vi "Extras.vi"(8 "Scope+Safety":T2={"Safety First"={"lim reset"=FALSE, "no limit"=FALSE, "pos slew rate * dt"=100, "neg slew rate * dt"=-100, "Count(Ticks)"=0}, "Scope IPs"={"Trigger Direction"=enum."minus-plus", "Trigger Delay (ms)"=0.0, "Aquisition Rate (kHz)"=4000.0, "Trigger Offset (V)"=0.0, "Scale Offset"={"Scaling"={"Error signal"=1, "Output"=1, "DC Monitor"=1, "Threshold"=1}, "Offset"={"Error Signal"=0, "Output"=0, "DC Monitor"=0, "Threshold"=0}}}}, 11 "Cavity Extras":T3={"Pre-Offset"={"OPO A"=0.0, "OPO B"=0.0, "MCC"=0.0, "Doubler"=0.0}, "Pre-Offset DC"={"OPO A"=0.0, "OPO B"=0.0, "MCC"=0.0, "Doubler"=0.0}, "I Max value"=20000, "I2 Max value"=20000, "Scan Offset"={"OPO A"=0.0, "OPO B"=0.0, "MCC"=0.0, "Doubler"=0.0}, "Scan Ampl."={"OPO A"=1000.0, "OPO B"=1000.0, "MCC"=1000.0, "Doubler"=1000.0}, "Scan-PII thresh"={"OPO A"=0, "OPO B"=0, "MCC"=0, "Doubler"=0}, "Re-Scan thresh"={"OPO A"=0, "OPO B"=0, "MCC"=0, "Doubler"=0}}) -> (0 "Extras Doubler":T1, 1 "Extras MCC":T1, 2 "Extras B":T1, 3 "Extras A":T1)   [LabVIEW 2010]
uses:
  Strict Type Defs/Cavity Extras.ctl
  Strict Type Defs/Pre-Offset.ctl
  Strict Type Defs/Scope and Safety.ctl
  Strict Type Defs/Extras PII.ctl
panel:
  in  "Extras PII":T1
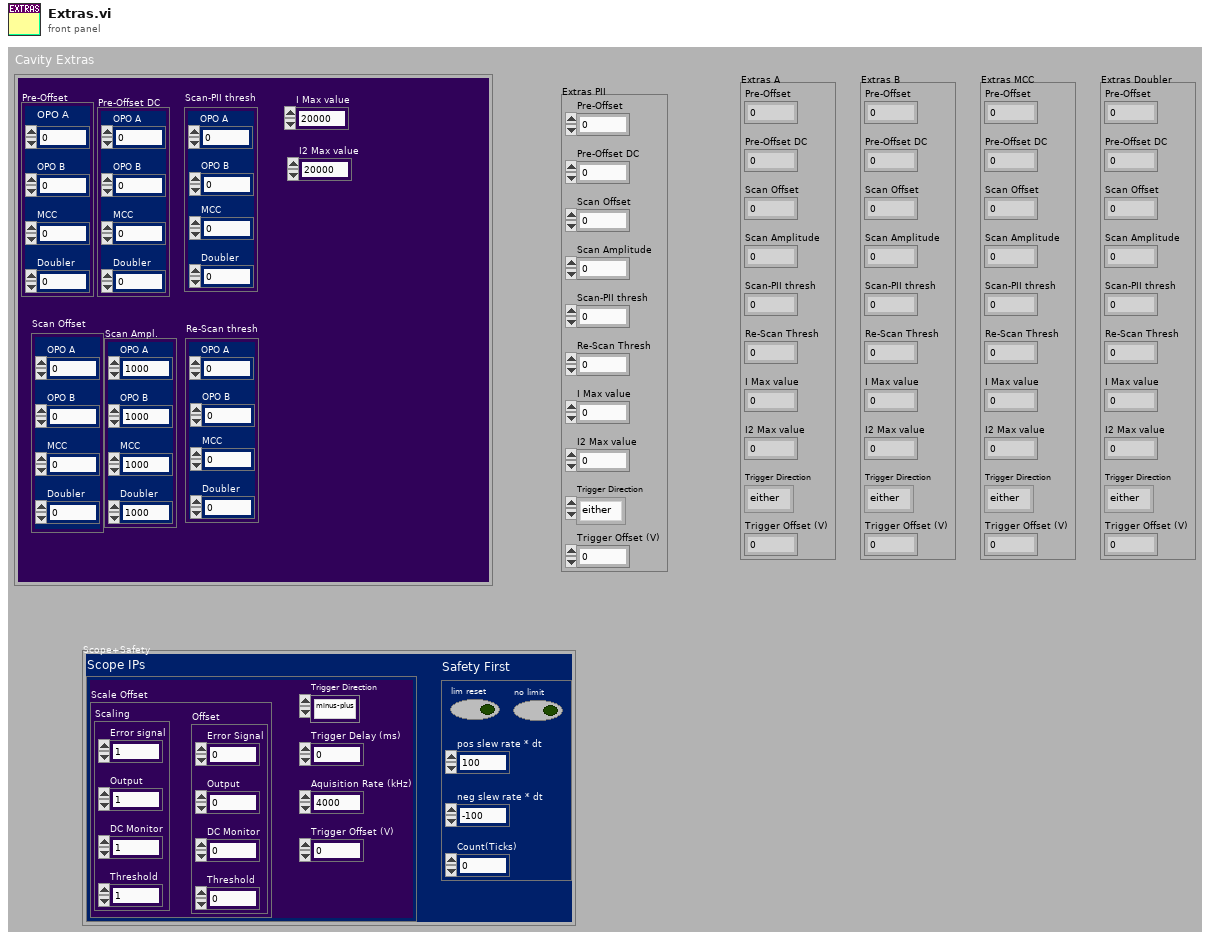
[diagram p1: front panel]
types:
  T1 = typedef "Extras PII.ctl" = cluster{"Pre-Offset":dbl, "Pre-Offset DC":dbl, "Scan Offset":dbl, "Scan Amplitude":dbl, "Scan-PII thresh":i16, "Re-Scan Thresh":i16, "I Max value":i32, "I2 Max value":i32, "Trigger Direction":enum8{"either", "minus-plus", "plus-minus"}, "Trigger Offset (V)":dbl}
  T2 = typedef "Scope and Safety.ctl" = cluster{"Safety First":cluster{"lim reset":bool, "no limit":bool, "pos slew rate * dt":i16, "neg slew rate * dt":i16, "Count(Ticks)":u32}, "Scope IPs":cluster{"Trigger Direction":enum8{"either", "minus-plus", "plus-minus"}, "Trigger Delay (ms)":dbl, "Aquisition Rate (kHz)":dbl, "Trigger Offset (V)":dbl, "Scale Offset":cluster{"Scaling":cluster{"Error signal":i16, "Output":i16, "DC Monitor":i16, "Threshold":i16}, "Offset":cluster{"Error Signal":i16, "Output":i16, "DC Monitor":i16, "Threshold":i16}}}}
  T3 = typedef "Cavity Extras.ctl" = cluster{"Pre-Offset":T4, "Pre-Offset DC":T4, "I Max value":i32, "I2 Max value":i32, "Scan Offset":T4, "Scan Ampl.":T4, "Scan-PII thresh":cluster{"OPO A":i16, "OPO B":i16, "MCC":i16, "Doubler":i16}, "Re-Scan thresh":cluster{"OPO A":i16, "OPO B":i16, "MCC":i16, "Doubler":i16}}
  T4 = typedef "Pre-Offset.ctl" = cluster{"OPO A":dbl, "OPO B":dbl, "MCC":dbl, "Doubler":dbl}
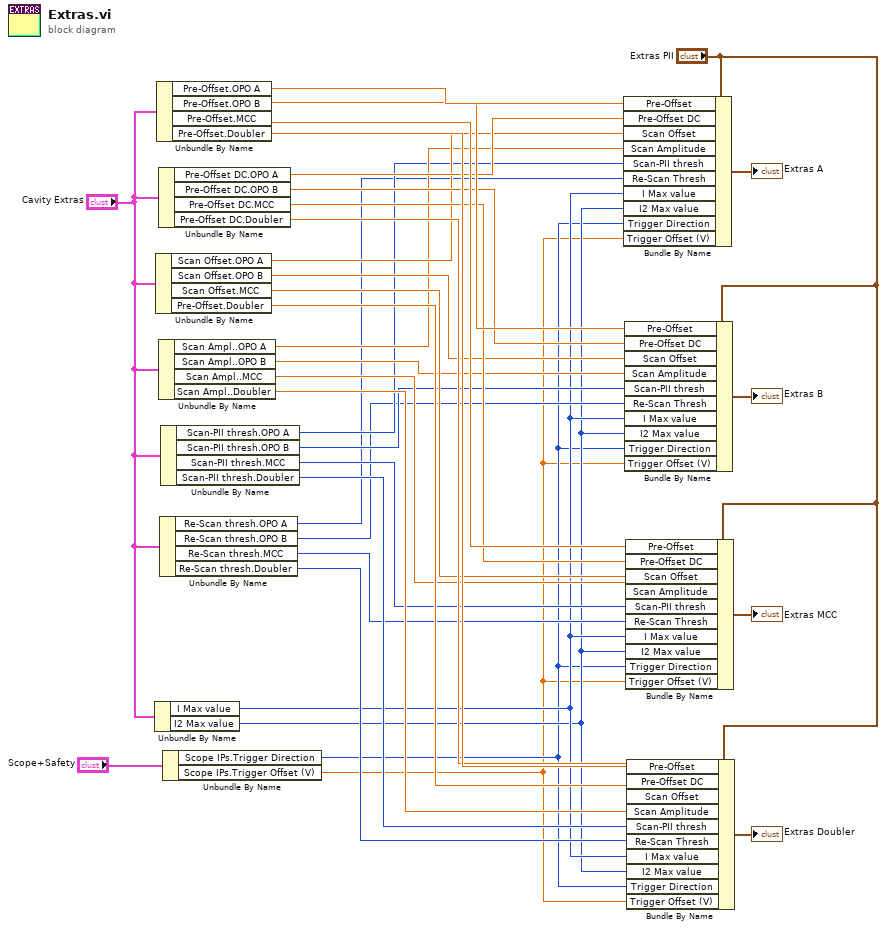
[diagram p0: block diagram]
diagram:
  n1 = Unbundle By Name("Cavity Extras") -> ("I Max value"=w4:i32, "I2 Max value"=w3:i32)
  n2 = Unbundle By Name("Cavity Extras") -> ("Scan Offset.OPO A"=w20:dbl, "Scan Offset.OPO B"=w19:dbl, "Scan Offset.MCC"=w18:dbl, "Pre-Offset.Doubler"=w17:dbl)
  n3 = Unbundle By Name("Cavity Extras") -> ("Pre-Offset.OPO A"=w28:dbl, "Pre-Offset.OPO B"=w27:dbl, "Pre-Offset.MCC"=w26:dbl, "Pre-Offset.Doubler"=w25:dbl)
  n4 = Unbundle By Name("Cavity Extras") -> ("Pre-Offset DC.OPO A"=w24:dbl, "Pre-Offset DC.OPO B"=w23:dbl, "Pre-Offset DC.MCC"=w22:dbl, "Pre-Offset DC.Doubler"=w21:dbl)
  n5 = Unbundle By Name("Cavity Extras") -> ("Scan Ampl..OPO A"=w16:dbl, "Scan Ampl..OPO B"=w15:dbl, "Scan Ampl..MCC"=w14:dbl, "Scan Ampl..Doubler"=w13:dbl)
  n6 = Unbundle By Name("Cavity Extras") -> ("Re-Scan thresh.OPO A"=w8:i16, "Re-Scan thresh.OPO B"=w7:i16, "Re-Scan thresh.MCC"=w6:i16, "Re-Scan thresh.Doubler"=w5:i16)
  n7 = Unbundle By Name("Cavity Extras") -> ("Scan-PII thresh.OPO A"=w12:i16, "Scan-PII thresh.OPO B"=w11:i16, "Scan-PII thresh.MCC"=w10:i16, "Scan-PII thresh.Doubler"=w9:i16)
  n8 = Unbundle By Name("Scope+Safety") -> ("Scope IPs.Trigger Direction"=w2:enum8{"either", "minus-plus", "plus-minus"}, "Scope IPs.Trigger Offset (V)"=w1:dbl)
  n9 = Bundle By Name(cluster="Extras PII", "Pre-Offset"=w28, "Pre-Offset DC"=w24, "Scan Offset"=w20, "Scan Amplitude"=w16, "Scan-PII thresh"=w12, "Re-Scan Thresh"=w8, "I Max value"=w4, "I2 Max value"=w3, "Trigger Direction"=w2, "Trigger Offset (V)"=w1) -> (→"Extras A":T1)
  n10 = Bundle By Name(cluster="Extras PII", "Pre-Offset"=w27, "Pre-Offset DC"=w23, "Scan Offset"=w19, "Scan Amplitude"=w15, "Scan-PII thresh"=w11, "Re-Scan Thresh"=w7, "I Max value"=w4, "I2 Max value"=w3, "Trigger Direction"=w2, "Trigger Offset (V)"=w1) -> (→"Extras B":T1)
  n11 = Bundle By Name(cluster="Extras PII", "Pre-Offset"=w26, "Pre-Offset DC"=w22, "Scan Offset"=w18, "Scan Amplitude"=w14, "Scan-PII thresh"=w10, "Re-Scan Thresh"=w6, "I Max value"=w4, "I2 Max value"=w3, "Trigger Direction"=w2, "Trigger Offset (V)"=w1) -> (→"Extras MCC":T1)
  n12 = Bundle By Name(cluster="Extras PII", "Pre-Offset"=w25, "Pre-Offset DC"=w21, "Scan Offset"=w17, "Scan Amplitude"=w13, "Scan-PII thresh"=w9, "Re-Scan Thresh"=w5, "I Max value"=w4, "I2 Max value"=w3, "Trigger Direction"=w2, "Trigger Offset (V)"=w1) -> (→"Extras Doubler":T1)
